vi "功能试验 总回转扭矩.vi"(9 "扭矩正转2":dbl[](array[numeric]), 10 "扭矩反转":dbl[](array[numeric]), 11 "扭矩正转1":dbl[](array[numeric])) -> (2 "扭矩反转平均值":dbl, 3 "扭矩正转平均值":dbl)   [LabVIEW 2015, in "Logging.lvlib"]
uses:
  Logging.lvlib
  <vilib>/Analysis/baseanly.llb/Mean (DBL).vi
  <vilib>/Analysis/NI_AALBase.lvlib
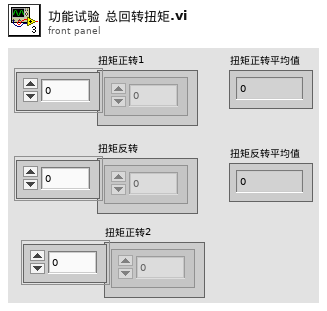
[diagram p1: front panel]
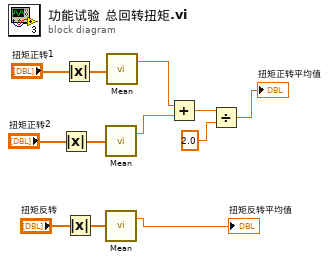
[diagram p0: block diagram]
diagram:
  n1 = Absolute Value(x="扭矩正转2") -> (abs(x)=w3:dbl[])
  n2 = Absolute Value(x="扭矩正转1") -> (abs(x)=w5:dbl[])
  n3 = Absolute Value(x="扭矩反转") -> (abs(x)=w1:dbl[])
  n4 = call-poly <vilib>:"Mean.vi"("X"=w3) -> ("mean"=w8:dbl)  [unwired: 1 out]
  n5 = call-poly <vilib>:"Mean.vi"("X"=w1) -> ("mean"=→"扭矩反转平均值":dbl)  [unwired: 1 out]
  n6 = call-poly <vilib>:"Mean.vi"("X"=w5) -> ("mean"=w9:dbl)  [unwired: 1 out]
  n7 = Add(x=w9, y=w8) -> (x+y=w12:dbl)
  n8 = Divide(x=w12, y=2.0) -> (x/y=→"扭矩正转平均值":dbl)
